vi "Configure.vi"(8 "error in (no error)":errorcluster, 11 "Template in":refnum<class "Cobolt.lvclass">=refnum) -> (0 "error out":errorcluster, 2 "cancelled?":bool, 3 "Template out":refnum<class "Cobolt.lvclass">)   [LabVIEW 2012, in "Cobolt.lvclass"]
doc: "The configure method configures the details for the RabbitMQ connection. \n\nIn the derived class, make a call to the parent for setting these parameters."
uses:
  Cobolt.lvclass
  <vilib>/Utility/miscctls.llb/LVPointTypeDef.ctl
panel:
  in  "Tab Control":enum32{"Comport", "Debug"}(tab)
  in  "VISA Wait":dbl[unit]=0.2
  in  "Enable Term Char":u16(ring) items=["Off", "On"]
  in  "Baud rate":u32=19200
  in  "parity":u16(ring) items=["None", "Odd", "Even", "Mark", "Space"]
  in  "stop bits":u16(ring)=10 items=["1.0"=10, "1.5"=15, "2.0"=20]
  in  "Flow control":u16(ring) items=["None"=0, "XON/XOFF"=1, "RTS/CTS"=2, "DTR/DSR"=4]
  in  "data bits":u16=8 min=5 max=8 step=1
  in  "VISA resource name":refnum<visa-resource-name>="COM1"
  in  "Time out":u32=2000
  in  "button:call parent":bool
  in  "button:ok":bool
  in  "button:cancel":bool
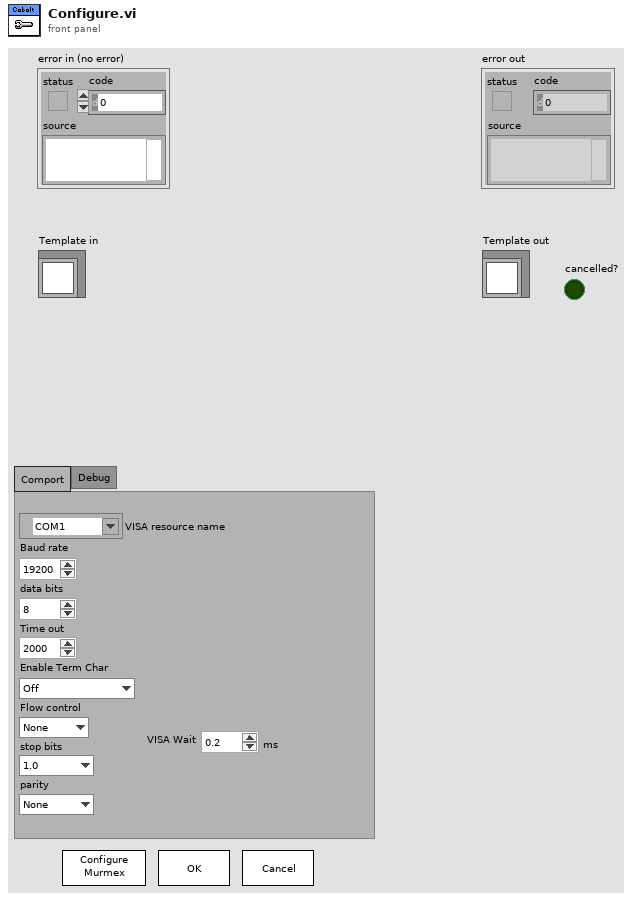
[diagram p1: front panel]
types:
  T1 = typedef "LVPointTypeDef.ctl" = cluster{"Horizontal":i16, "Vertical":i16}
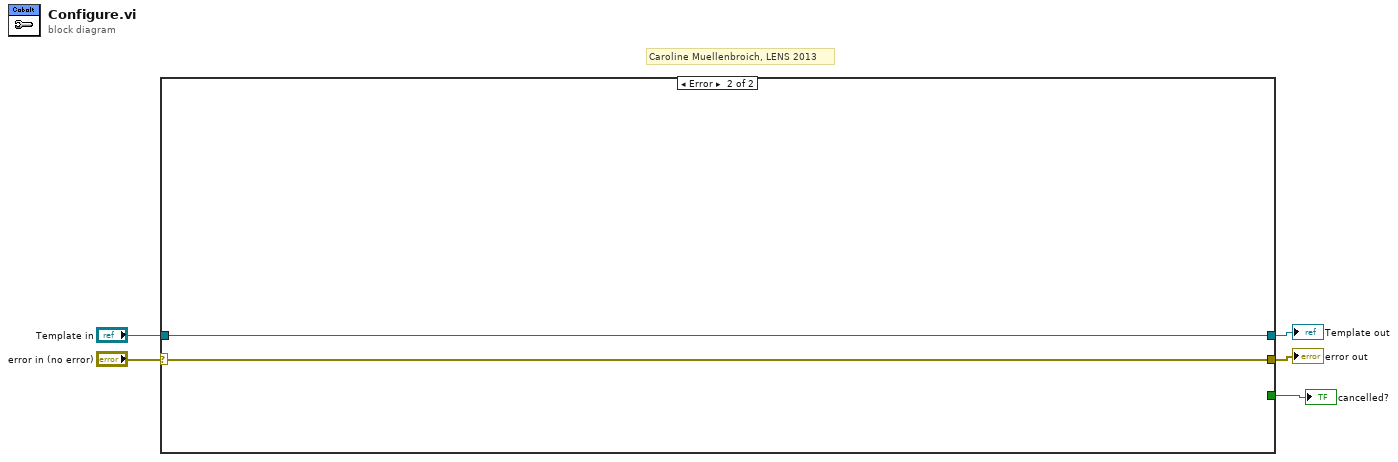
[diagram p0: block diagram]
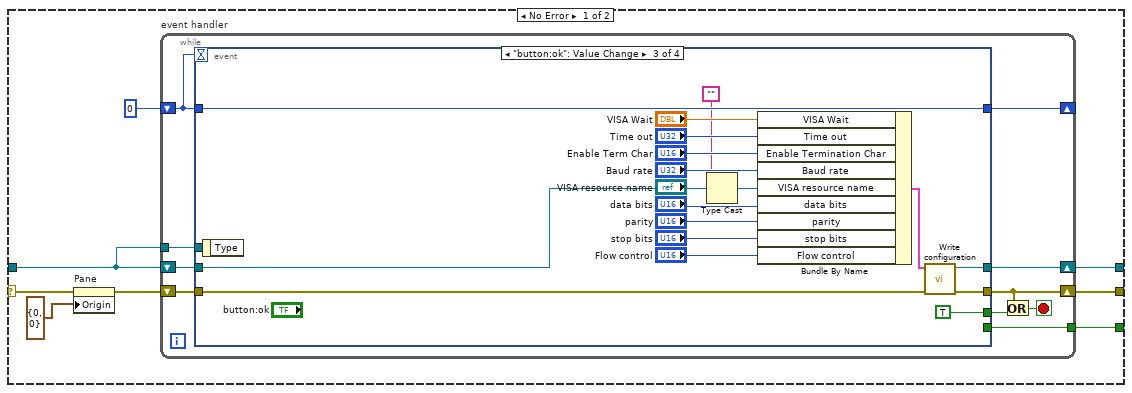
[diagram p2: hidden frame]
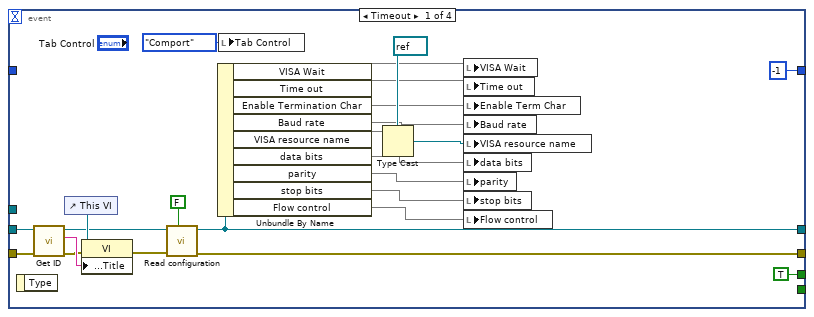
[diagram p3: hidden frame]
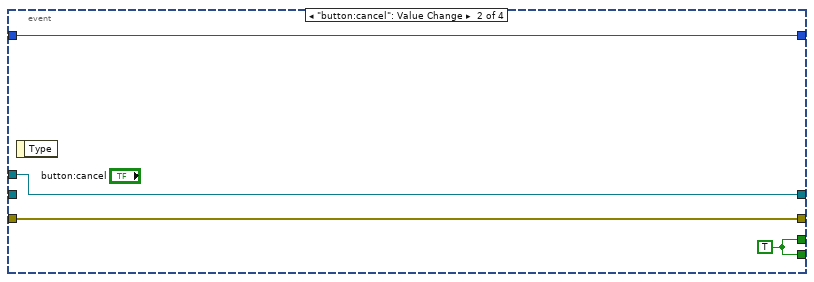
[diagram p4: hidden frame]
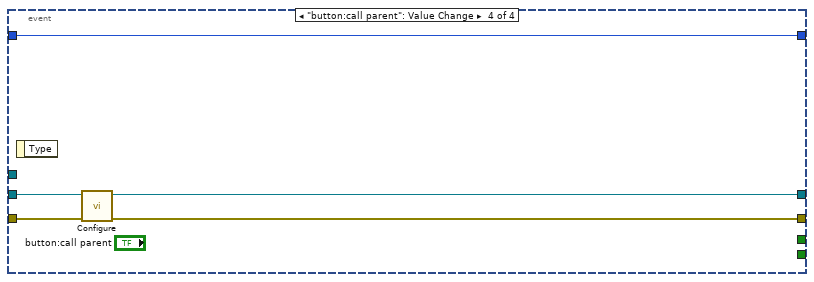
[diagram p5: hidden frame]
diagram:
  # "Caroline Muellenbroich, LENS 2013"
  n1 = case shown="Error" "error in (no error)" {
    selector: "error in (no error)" -> [w11 w76]
    tunnel: "Template in" -> [w9 w75]
    tunnel: [w8 w75] -> w3
    tunnel: [w7 w76] -> w2
    tunnel: [w6 _] -> w1
    frame No Error {
      n2 = property on="Pane" class="Pane"(error in=w11, "Origin"=T1 {"Horizontal"=0, "Vertical"=0}) -> (error out=w10:errorcluster)  [unwired: 1 in, 1 out]
      n3 = while "event handler" {
        tunnel: [w23] -> w6
        shift-right: [w22] -> w8
        shift-left: w9 -> [w14]
        shift-right: [w20] -> w7
        shift-left: w10 -> [w21]
        shift-right: [w17] -> _
        shift-left: 0 -> [w16]
        tunnel: w9 -> [w15]
        stop <- w18 stop-if-true
        n4 = event shown="[2] \"button:ok\": Value Change" {
          selector: _ -> [_ _ _ _]
          dyn-events: _ -> [_ _ _ _]
          timeout: w16 -> [_ _ _ _]
          tunnel: [w47 w50 w64 w72] -> w20
          tunnel: [_ w49 _ _] -> w23
          tunnel: [w45 w51 w66 w71] -> w22
          tunnel: w21 -> [w40 w50 w65 w73]
          tunnel: w14 -> [w39 _ w68 w74]
          tunnel: w15 -> [_ w51 _ _]
          tunnel: [TRUE ("cancelled?") w49 TRUE ("cancelled?") _] -> w19
          tunnel: [-1 w48 w63 w70] -> w17
          tunnel: w16 -> [_ w48 w63 w70]
          event Timeout {
            n5 = event-data() -> ()  [unwired: 1 in, 1 out]
            n6 = call "Get ID.vi"("error in (no error)"=w40, "Murmex in"=w39) -> ("error out"=w42:errorcluster, "component id"=w43:string, "Murmex out"=w38:refnum<class "Cobolt.lvclass">)  [unwired: 7 in]
            n7 = control-ref of="This VI"() -> (w41:refnum<vi>)
            n8 = property class="VI"(reference=w41, error in=w42, "Front Panel.Title"=w43) -> (error out=w37:errorcluster)  [unwired: 1 out]
            n9 = call-dynamic "Read configuration.vi"("force loading?"=FALSE, "error in (no error)"=w37, "Template in"=w38) -> ("error out"=w47:errorcluster, "Template out"=w45:refnum<class "Cobolt.lvclass">)  [unwired: 7 in]
            n10 = Unbundle By Name(w45) -> ("VISA Wait"=w32, "Time out"=w31, "Enable Termination Char"=w30, "Baud rate"=w29, "VISA resource name"=w36, "data bits"=w27, "parity"=w26, "stop bits"=w25, "Flow control"=w24)
            n11 = local write "Tab Control"(enum32{"Comport", "Debug"}."Comport" ("Tab Control")) -> ()
            n12 = Type Cast(type=refnum<visa-resource-name> refnum ("VISA resource name"), x=w36) -> (*(type *) &x=w28:refnum<visa-resource-name>)
            n13 = local write "VISA Wait"(w32) -> ()
            n14 = local write "Time out"(w31) -> ()
            n15 = local write "Enable Term Char"(w30) -> ()
            n16 = local write "Baud rate"(w29) -> ()
            n17 = local write "VISA resource name"(w28) -> ()
            n18 = local write "data bits"(w27) -> ()
            n19 = local write "parity"(w26) -> ()
            n20 = local write "stop bits"(w25) -> ()
            n21 = local write "Flow control"(w24) -> ()
          }
          event "button:cancel": Value Change {
            w49 = TRUE ("cancelled?")
            n22 = event-data() -> ()  [unwired: 1 in, 1 out]
          }
          event "button:ok": Value Change {
            n23 = event-data() -> ()  [unwired: 1 in, 1 out]
            n24 = Type Cast(type="", x="VISA resource name") -> (*(type *) &x=w58:string)
            n25 = Bundle By Name(cluster=w68, "VISA Wait"="VISA Wait", "Time out"="Time out", "Enable Termination Char"="Enable Term Char", "Baud rate"="Baud rate", "VISA resource name"=w58, "data bits"="data bits", "parity"="parity", "stop bits"="stop bits", "Flow control"="Flow control") -> (w67:cluster{})
            n26 = call-dynamic "Write configuration.vi"("error in (no error)"=w65, "Template in"=w67) -> ("error out"=w64:errorcluster, "Template out"=w66:refnum<class "Cobolt.lvclass">)  [unwired: 8 in]
          }
          event "button:call parent": Value Change {
            n27 = event-data() -> ()  [unwired: 1 in, 1 out]
            n28 = call-parent "Configure.vi"("error in (no error)"=w73, "Murmex in"=w74) -> ("error out"=w72:errorcluster, "Murmex out"=w71:refnum<class "Cobolt.lvclass">)  [unwired: 7 in, 1 out]
          }
        }
        n29 = Or(x=w20, y=w19) -> (x .or. y?=w18:bool)
      }
    }
    frame Error {
    }
  }
  "error out" <- w2
  "Template out" <- w3
  "cancelled?" <- w1
